vi "Get Client Certificate (Client).vi"(10 "Client Certificates":T1) -> (2 "client certificate file":path)   [LabVIEW 2013, in "OPC UA runtime.lvclass"]
doc: "Get client certificate used to create an OPC UA client connection"
uses:
  OPC UA runtime.lvclass
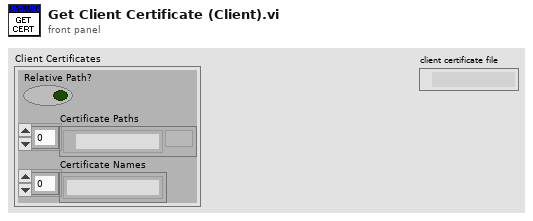
[diagram p1: front panel]
types:
  T1 = cluster{"Relative Path?":bool, "Certificate Paths":path[], "Certificate Names":string[]}
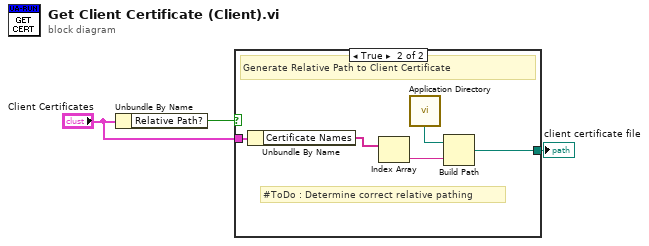
[diagram p0: block diagram]
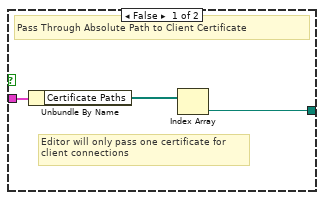
[diagram p2: hidden frame]
diagram:
  n1 = Unbundle By Name("Client Certificates") -> ("Relative Path?"=w3:bool)
  n2 = case shown="True" w3 {
    tunnel: "Client Certificates" -> [w6 w11]
    tunnel: [w4 w7] -> w1
    frame False {
      # "Editor will only pass one certificate for\nclient connections"
      # "Pass Through Absolute Path to Client Certificate"
      n3 = Unbundle By Name(w6) -> ("Certificate Paths"=w5:path[])
      n4 = Index Array(array=w5) -> (element=w4:path)  [unwired: 1 in]
    }
    frame True {
      # "#ToDo : Determine correct relative pathing"
      # "Generate Relative Path to Client Certificate"
      n5 = Unbundle By Name(w11) -> ("Certificate Names"=w10:string[])
      n6 = Index Array(array=w10) -> (element=w9:string)  [unwired: 1 in]
      n7 = call <vilib>:"Application Directory.vi"() -> ("Application Directory"=w8:path)
      n8 = Build Path(base path=w8, name or relative path=w9) -> (appended path=w7:path)
    }
  }
  "client certificate file" <- w1
